vi "Write_Parameters.vi"(8 "error in (no error)":errorcluster, 9 "Param Controls":T1 {"Control Reference\nVoltage (MV)" min=0.3 max=3.0 step=0.1; "High Voltage\nPS Setting (kV)" min=0.0 max=18.0 step=0.2; "Spark\nLimit" min=0.0 max=10.0 step=1.0}, 11 "AccelNET.lvlib:TCP.lvclass":refnum<class "TCP.lvclass">) -> (0 "Error Out":errorcluster)   [LabVIEW 2012, in "AccelNET.lvlib" / "TCP.lvclass"]
uses:
  TCP.lvclass
  Parameters_Control.ctl
  Useful_SubVIs.lvlib
  Useful_Controls.lvlib
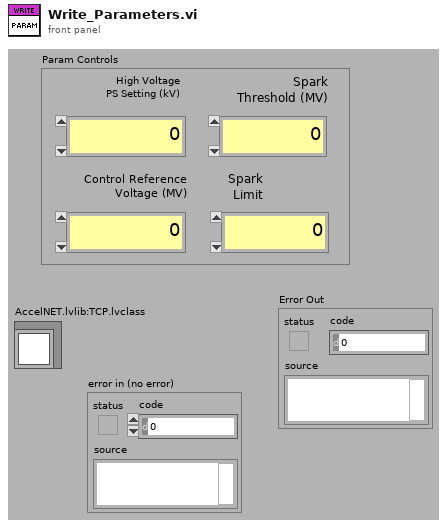
[diagram p1: front panel]
types:
  T1 = typedef "AccelNET.lvlib/Useful_Controls.lvlib/Parameters_Control.ctl" = cluster{"Spark\nThreshold (MV)":dbl, "Spark\nLimit":dbl, "High Voltage\nPS Setting (kV)":dbl, "Control Reference\nVoltage (MV)":dbl}
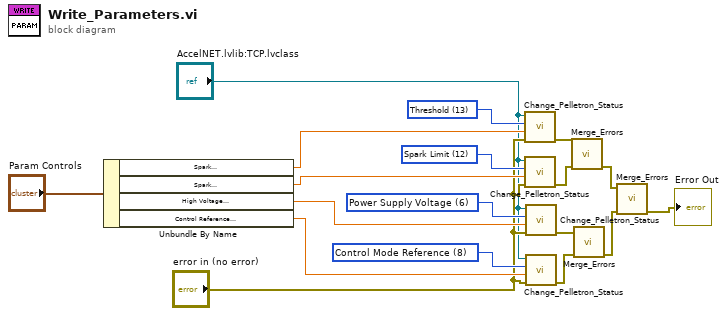
[diagram p0: block diagram]
diagram:
  w14 = u16 13 items=["GV", "Blower", "Main Power Supply", "Chain Power Supply", "Chain", "Rotating Shaft", "Power Supply Voltage", "Control Mode", "Control Mode Reference", "Chain Bypass", "Rotating Shaft Bypass", "Spark Counter", "Spark Limit", "Threshold", "Spark Counter Reset", "Ion Filament"] ("Write Selector")
  w15 = u16 12 items=["GV", "Blower", "Main Power Supply", "Chain Power Supply", "Chain", "Rotating Shaft", "Power Supply Voltage", "Control Mode", "Control Mode Reference", "Chain Bypass", "Rotating Shaft Bypass", "Spark Counter", "Spark Limit", "Threshold", "Spark Counter Reset", "Ion Filament"] ("Write Selector")
  w16 = u16 6 items=["GV", "Blower", "Main Power Supply", "Chain Power Supply", "Chain", "Rotating Shaft", "Power Supply Voltage", "Control Mode", "Control Mode Reference", "Chain Bypass", "Rotating Shaft Bypass", "Spark Counter", "Spark Limit", "Threshold", "Spark Counter Reset", "Ion Filament"] ("Write Selector")
  w17 = u16 8 items=["GV", "Blower", "Main Power Supply", "Chain Power Supply", "Chain", "Rotating Shaft", "Power Supply Voltage", "Control Mode", "Control Mode Reference", "Chain Bypass", "Rotating Shaft Bypass", "Spark Counter", "Spark Limit", "Threshold", "Spark Counter Reset", "Ion Filament"] ("Write Selector")
  n1 = Unbundle By Name("Param Controls") -> ("Spark\nThreshold (MV)"=w10:dbl, "Spark\nLimit"=w11:dbl, "High Voltage\nPS Setting (kV)"=w12:dbl, "Control Reference\nVoltage (MV)"=w13:dbl)
  n2 = call "Change_Pelletron_Status.vi"("error in (no error)"="error in (no error)", "Write Value"=w10, "Write Selector"=w14, "AccelNET.lvlib:TCP.lvclass"="AccelNET.lvlib:TCP.lvclass") -> ("error out"=w9:errorcluster)  [unwired: 7 in]
  n3 = call "Change_Pelletron_Status.vi"("error in (no error)"="error in (no error)", "Write Value"=w11, "Write Selector"=w15, "AccelNET.lvlib:TCP.lvclass"="AccelNET.lvlib:TCP.lvclass") -> ("error out"=w8:errorcluster)  [unwired: 7 in]
  n4 = call "Change_Pelletron_Status.vi"("error in (no error)"="error in (no error)", "Write Value"=w12, "Write Selector"=w16, "AccelNET.lvlib:TCP.lvclass"="AccelNET.lvlib:TCP.lvclass") -> ("error out"=w7:errorcluster)  [unwired: 7 in]
  n5 = call "Change_Pelletron_Status.vi"("error in (no error)"="error in (no error)", "Write Value"=w13, "Write Selector"=w17, "AccelNET.lvlib:TCP.lvclass"="AccelNET.lvlib:TCP.lvclass") -> ("error out"=w1:errorcluster)  [unwired: 7 in]
  n6 = call "Merge_Errors.vi"("Error 2"=w8, "Error 1"=w9) -> ("Error Out"=w5:errorcluster)  [unwired: 9 in]
  n7 = call "Merge_Errors.vi"("Error 2"=w1, "Error 1"=w7) -> ("Error Out"=w6:errorcluster)  [unwired: 9 in]
  n8 = call "Merge_Errors.vi"("Error 2"=w6, "Error 1"=w5) -> ("Error Out"=→"Error Out":errorcluster)  [unwired: 9 in]
